vi "ErrorHandling.vi"(8 "error in (no error)":errorcluster, 10 "Vi-name":string) -> (0 "error out":errorcluster)   [LabVIEW 2015]
uses:
  <vilib>/Utility/error.llb/DialogType.ctl
types:
  T1 = typedef "DialogType.ctl" = u16
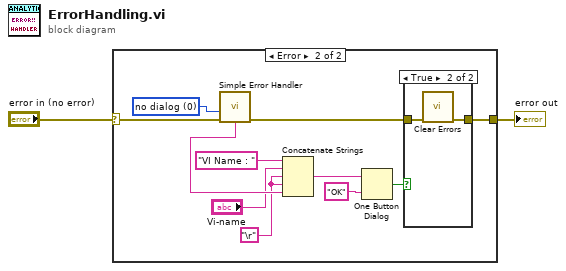
[diagram p0: block diagram]
diagram:
  n1 = case shown="Error" "error in (no error)" {
    selector: "error in (no error)" -> [w3 w5]
    tunnel: [w3 w6] -> w2
    frame No Error {
    }
    frame Error {
      w10 = "\r"
      w14 = T1 0 items=["no dialog", "OK message", "continue or stop message", "OK message + warnings", "continue/stop + warnings"] ("type of dialog (OK msg:1)")
      n2 = call <vilib>:"Simple Error Handler.vi"("type of dialog (OK msg:1)"=w14, "error in (no error)"=w5) -> ("error out"=w7:errorcluster, "message"=w12:string)  [unwired: 3 in, 3 out]
      n3 = Concatenate Strings("VI Name : " ("Vi-name"), "Vi-name", w10, w10, w12) -> (w11:string)
      n4 = One Button Dialog(message=w11, button name ("OK")="OK") -> (true=w8:bool)
      n5 = case shown="True" w8 {
        tunnel: w7 -> [w15 w17]
        tunnel: [w15 w16] -> w6
        frame False {
        }
        frame True {
          n6 = call <vilib>:"Clear Errors.vi"("error in (no error)"=w17) -> ("error out"=w16:errorcluster)  [unwired: 5 in, 1 out]
        }
      }
    }
  }
  "error out" <- w2
